vi "generic_reply_extract.vi"(5 "multipart message in":string[](array[string]), 11 "error in (no error)":errorcluster) -> (3 "Valid Message?":bool, 6 "Mode":enum16{"RF", "IF", "BB"}(ring), 14 "Debug info":string, 15 "error out":errorcluster)   [LabVIEW 2019, in "mmW_commands.lvlib"]
uses:
  mmW_commands.lvlib
  TypeDefs/commands.ctl
  commands/_depr_initialize_hw.ctl
  reply_statuscode.ctl
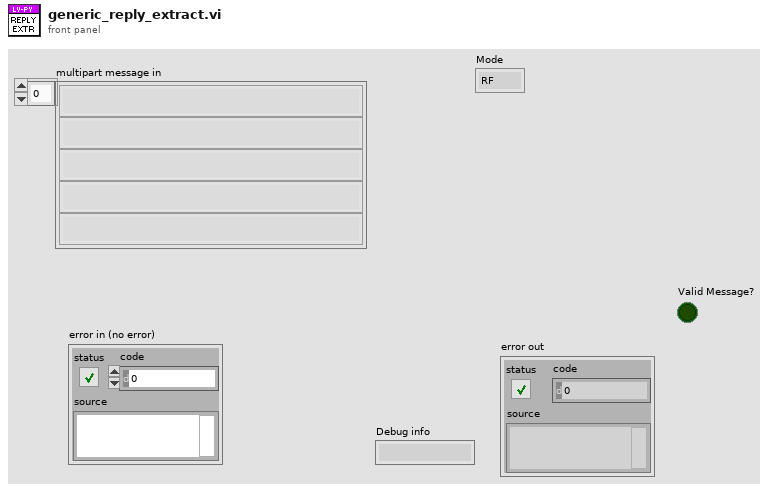
[diagram p1: front panel]
types:
  T1 = typedef "mmW_commands.lvlib/commands.ctl" = enum16{"configure_fs", "configure_rf", "configure_trigger", "equalization_enable", "equalization_start", "lo_sync_enable", "equalization_stop", "get_instrument_status", "get_versions", "initialize_hw", "pop_rx", "set_log_level", "Shutdown", "start", "start_instrument_app", "stop", "transceive", "trigger_burst", "trigger_sync_enable", "Write TX", "resp_generic", "resp_waveform"}
  T2 = typedef "mmW_commands.lvlib/_depr_initialize_hw.ctl" = cluster{"mode":enum16{"RF", "IF", "BB"}, "hwclass":string}
  T3 = typedef "mmW_commands.lvlib/reply_statuscode.ctl" = enum16{"Error", "OK"}
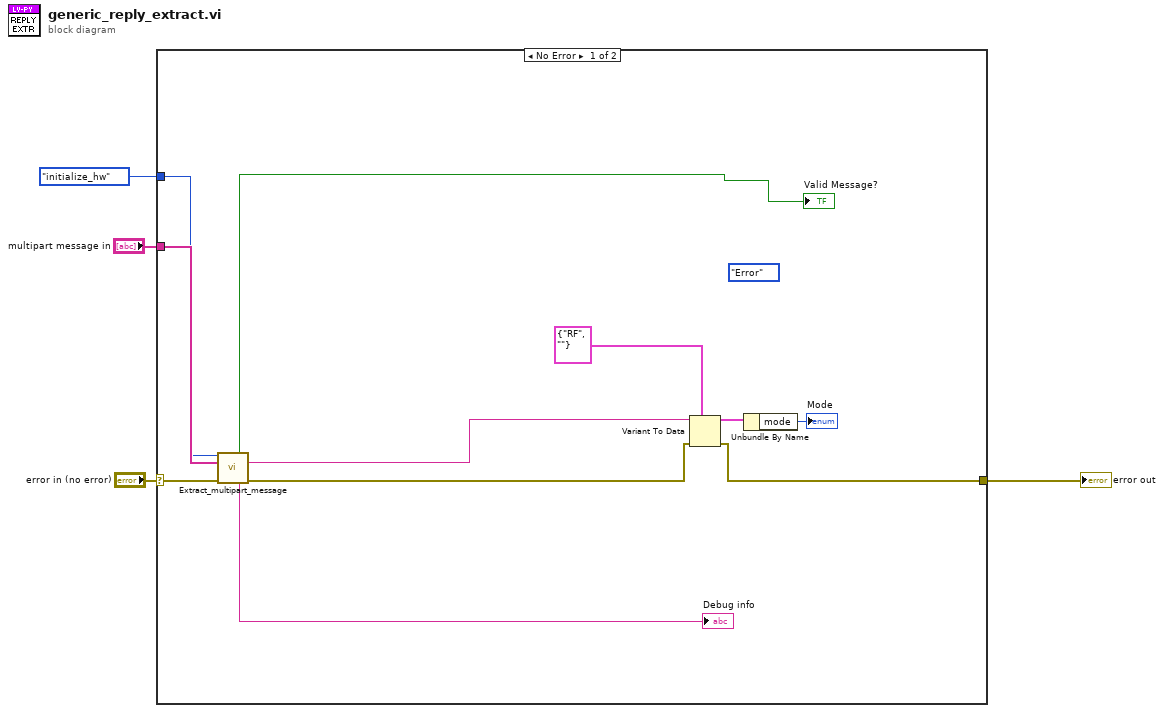
[diagram p0: block diagram]
diagram:
  n1 = case shown="No Error" "error in (no error)" {
    selector: "error in (no error)" -> [w15 w16]
    tunnel: [w11 w16] -> w4
    tunnel: "multipart message in" -> [w14 _]
    tunnel: commands."initialize_hw" ("mmW_instrument_commands") -> [w10 _]
    frame No Error {
      (unwired) reply_statuscode."Error" ("Enum")
      n2 = call "Extract_multipart_message.vi"("multipart message in"=w10, 5:w14, "error in (no error)"=w15) -> ("Valid message?"=→"Valid Message?":bool, "parameters"=w12:string, "Debug info"=→"Debug info":string, "error out"=w13:errorcluster)  [unwired: 5 in, 4 out]
      n3 = Variant To Data(error in=w13, type=T2 {"mode"=enum."RF", "hwclass"=""} ("Cluster"), Variant=w12) -> (data=w6:T2, error out=w11:errorcluster)
      n4 = Unbundle By Name(w6) -> ("mode"=→"Mode":enum16{"RF", "IF", "BB"})
    }
    frame Error {
    }
  }
  "error out" <- w4
